vi "move_invader.vi"(1 "MainCluster_IN":T11) -> (0 "MainCluster_OUT":T11)   [LabVIEW 2022 SP3]
uses:
  InitCluster.ctl
  CharacterCluster.ctl
  <vilib>/picture/picture.llb/imagedata.ctl
  ShotInitCluster.ctl
  <vilib>/Utility/miscctls.llb/LVPositionTypeDef.ctl
  <vilib>/Utility/miscctls.llb/LVBoundsTypeDef.ctl
  ShotCluster.ctl
  move_dir_ud.ctl
  InvaderPositionArray.ctl
  move_dir_lr.ctl
  Globals.vi
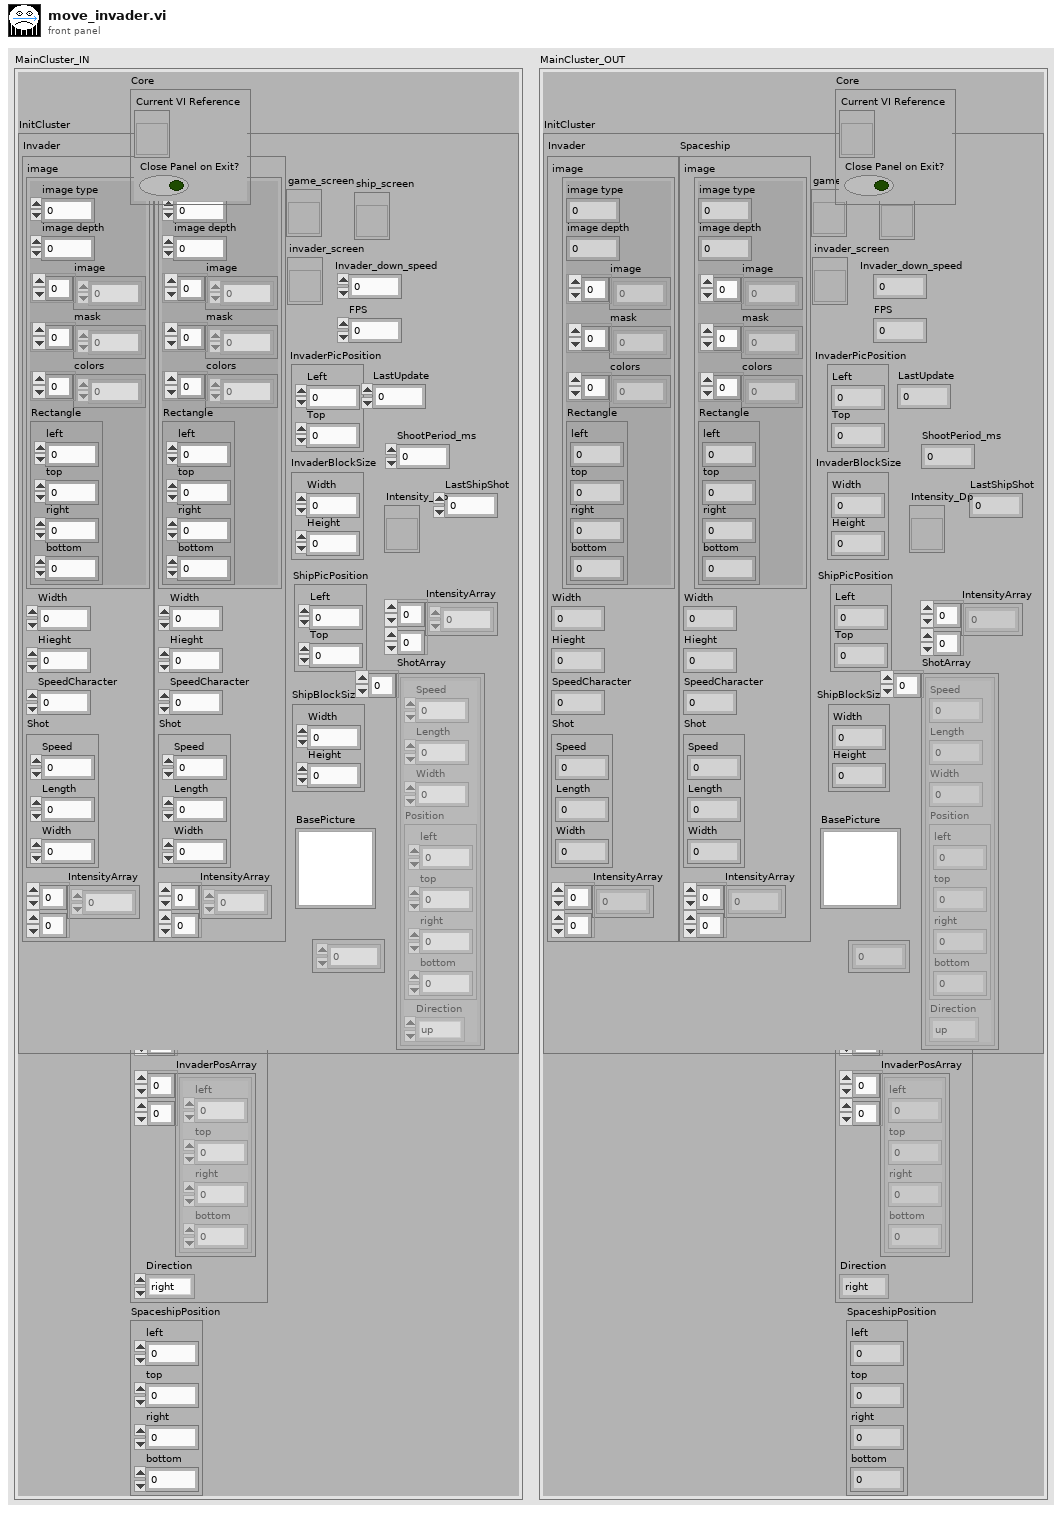
[diagram p1: front panel]
types:
  T1 = typedef "InitCluster.ctl" = cluster{"Invader":T2, "Spaceship":T2, "game_screen":refnum<vi>, "BasePicture":picture, "invader_screen":refnum<vi>, "InvaderPicPosition":T5, "Invader_down_speed":i16, "FPS":u16, "InvaderBlockSize":T6, "ship_screen":refnum<vi>, "ShipBlockSize":T6, "ShipPicPosition":T5, "LastUpdate":u32, "Intensity_Dp":refnum<vi>, "IntensityArray":u8[][], "ShotArray":T7[], "InvaderShotTimeArray":u32[], "ShootPeriod_ms":i32, "LastShipShot":u32}
  T2 = typedef "CharacterCluster.ctl" = cluster{"image":T3, "Width":u32, "Hieght":u32, "SpeedCharacter":u32, "Shot":T4, "IntensityArray":u8[][]}
  T3 = typedef "imagedata.ctl" = cluster{"image type":i32, "image depth":i32, "image":u8[], "mask":u8[], "colors":u32[], "Rectangle":cluster{"left":i16, "top":i16, "right":i16, "bottom":i16}}
  T4 = typedef "ShotInitCluster.ctl" = cluster{"Speed":u32, "Length":u32, "Width":u32}
  T5 = typedef "LVPositionTypeDef.ctl" = cluster{"Left":i32, "Top":i32}
  T6 = typedef "LVBoundsTypeDef.ctl" = cluster{"Width":u32, "Height":u32}
  T7 = typedef "ShotCluster.ctl" = cluster{"Speed":u32, "Length":u32, "Width":u32, "Position":cluster{"left":i16, "top":i16, "right":i16, "bottom":i16}, "Direction":T8}
  T8 = typedef "move_dir_ud.ctl" = enum16{"up", "down"}
  T9 = typedef "InvaderPositionArray.ctl" = cluster{"InvaderAlive":bool[][], "InvaderPosArray":cluster{"left":i16, "top":i16, "right":i16, "bottom":i16}[][], "Direction":T10}
  T10 = typedef "move_dir_lr.ctl" = enum16{"right", "left"}
  T11 = cluster{"Core":cluster{"Current VI Reference":refnum<vi>, "Close Panel on Exit?":bool}, "InitCluster":T1, "InvaderPosArray":T9, "SpaceshipPosition":cluster{"left":i16, "top":i16, "right":i16, "bottom":i16}}
  T12 = cluster{"left":i16, "top":i16, "right":i16, "bottom":i16}[][]
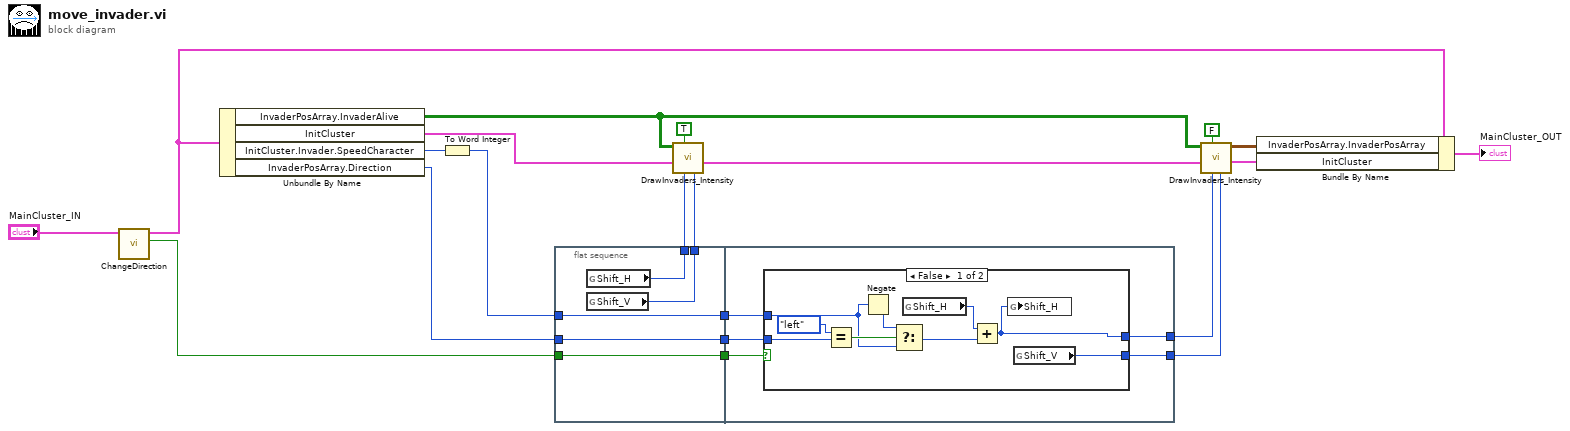
[diagram p0: block diagram]
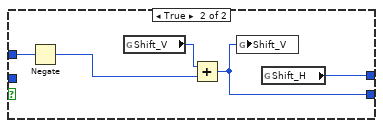
[diagram p2: hidden frame]
diagram:
  n1 = call "ChangeDirection.vi"("MainCluster_IN"="MainCluster_IN") -> ("DirectionChanged"=w12:bool, "MainCluster_OUT"=w15:T11)  [unwired: 9 in]
  n2 = Unbundle By Name(w15) -> ("InvaderPosArray.InvaderAlive"=w11:bool[][], "InitCluster"=w10:T1, "InitCluster.Invader.SpeedCharacter"=w20:u32, "InvaderPosArray.Direction"=w17:T10)
  n3 = To Word Integer(number=w20) -> (16bit integer=w16:i16)
  n4 = flat-sequence {
    tunnel: w12 -> [w24]
    tunnel: w16 -> [w25]
    tunnel: w17 -> [w26]
    tunnel: [w26] -> w8
    tunnel: [w25] -> w7
    tunnel: [w24] -> w6
    tunnel: [w23] -> w5
    tunnel: [w22] -> w4
    tunnel: [w29] -> w14
    tunnel: [w28] -> w13
    tunnel: w8 -> [w31]
    tunnel: w7 -> [w30]
    tunnel: w6 -> [w27]
    frame #0 {
      n5 = global read "Globals.vi" "Shift_H"() -> (w23:i16)
      n6 = global read "Globals.vi" "Shift_V"() -> (w22:i16)
    }
    frame #1 {
      n7 = case shown="False" w27 {
        tunnel: w31 -> [w38 _]
        tunnel: w30 -> [w36 w45]
        tunnel: [w33 w41] -> w29
        tunnel: [w32 w42] -> w28
        frame False {
          n8 = Equal?(x=move_dir_lr."left" ("Direction"), y=w38) -> (x = y?=w39:bool)
          n9 = Negate(x=w36) -> (-x=w37:i16)
          n10 = Select(t=w37, s=w39, f=w36) -> (s? t:f=w34:i16)
          n11 = global read "Globals.vi" "Shift_H"() -> (w35:i16)
          n12 = Add(x=w35, y=w34) -> (x+y=w33:i16)
          n13 = global write "Globals.vi" "Shift_H"(w33) -> ()
          n14 = global read "Globals.vi" "Shift_V"() -> (w32:i16)
        }
        frame True {
          n15 = Negate(x=w45) -> (-x=w43:i16)
          n16 = global read "Globals.vi" "Shift_V"() -> (w44:i16)
          n17 = Add(x=w44, y=w43) -> (x+y=w42:i16)
          n18 = global write "Globals.vi" "Shift_V"(w42) -> ()
          n19 = global read "Globals.vi" "Shift_H"() -> (w41:i16)
        }
      }
    }
  }
  n20 = call "DrawInvaders_Intensity.vi"("Step_V"=w4, "Step_H"=w5, "Clear"=TRUE, "InitCluster_IN"=w10, "InvaderArray"=w11) -> ("InitCluster_OUT"=w9:T1)  [unwired: 5 in, 1 out]
  n21 = call "DrawInvaders_Intensity.vi"("Step_V"=w13, "Step_H"=w14, "Clear"=FALSE, "InitCluster_IN"=w9, "InvaderArray"=w11) -> ("InitCluster_OUT"=w1:T1, "InvaderPosArray"=w18:T12)  [unwired: 5 in]
  n22 = Bundle By Name(cluster=w15, "InvaderPosArray.InvaderPosArray"=w18, "InitCluster"=w1) -> (→"MainCluster_OUT":T11)
